vi "subBuildXYGraph.vi"(7 "Enable":bool=TRUE, 8 "error in (no error)":errorcluster, 9 "Reset":bool, 10 "Y Input":dynamicdata(waveform), 11 "X Input":dynamicdata(waveform)) -> (0 "error out":errorcluster, 2 "XY Graph":cluster{"X":dbl[], "Y":dbl[]}[](array[cluster]))   [LabVIEW 2020]
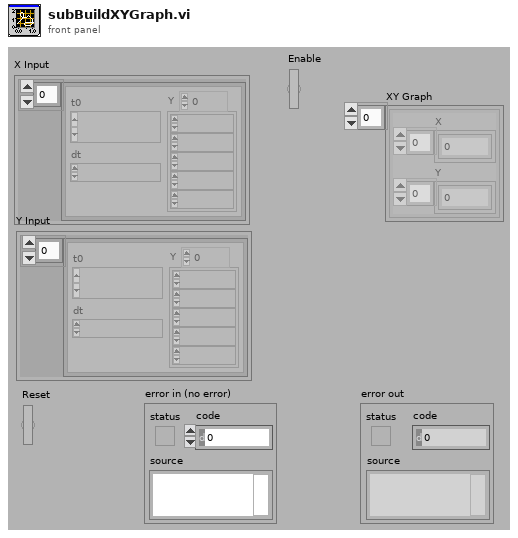
[diagram p1: front panel]
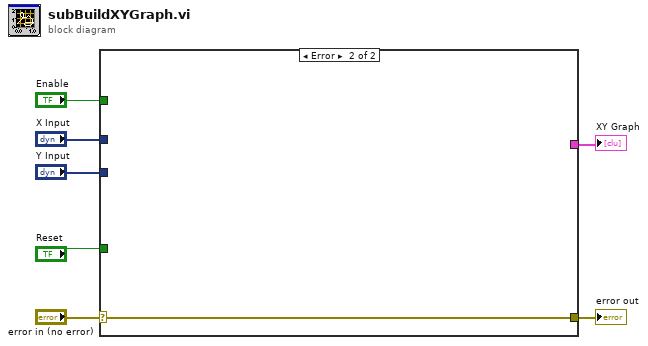
[diagram p0: block diagram]
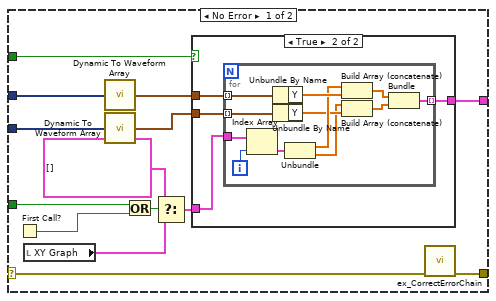
[diagram p2: hidden frame]
diagram:
  n1 = case shown="Error" "error in (no error)" {
    selector: "error in (no error)" -> [w9 w39]
    tunnel: [w21 _] -> w7
    tunnel: "Enable" -> [w18 _]
    tunnel: "Reset" -> [w16 _]
    tunnel: "Y Input" -> [w12 _]
    tunnel: "X Input" -> [w11 _]
    tunnel: [w10 w39] -> w1
    frame No Error {
      n2 = First Call?() -> (First Call?: T/F=w15:bool)
      n3 = local read "XY Graph"() -> (w8:cluster{"X":dbl[], "Y":dbl[]}[])
      n4 = call "Dynamic To Waveform Array.vi"("Input"=w11) -> ("Output"=w14:waveform(dbl)[])  [unwired: 4 out]
      n5 = call "Dynamic To Waveform Array.vi"("Input"=w12) -> ("Output"=w13:waveform(dbl)[])  [unwired: 4 out]
      n6 = Or(x=w16, y=w15) -> (x .or. y?=w17:bool)
      n7 = Select(t=cluster{"Y":dbl[], "Y":dbl[]}[] [] ("Output Array"), s=w17, f=w8) -> (s? t:f=w19:cluster{"X":dbl[], "Y":dbl[]}[])
      n8 = case shown="True" w18 {
        tunnel: [w22 w26] -> w21
        tunnel: w14 -> [_ w24]
        tunnel: w13 -> [_ w23]
        tunnel: w19 -> [w22 w25]
        frame False {
        }
        frame True {
          n9 = for {
            tunnel: [w38] -> w26 mode=indexing
            tunnel: w24 -> [w27] mode=indexing
            tunnel: w23 -> [w28] mode=indexing
            tunnel: w25 -> [w31]
            i -> [w29]
            n10 = Index Array(array=w31, index=w29) -> (element=w30:cluster{"X":dbl[], "Y":dbl[]})
            n11 = Unbundle By Name(w27) -> ("Y"=w37:dbl[])
            n12 = Unbundle By Name(w28) -> ("Y"=w34:dbl[])
            n13 = Unbundle(w30) -> ("X"=w35:dbl[], "Y"=w33:dbl[])
            n14 = Build Array (concatenate)(w35, w37) -> (w36:dbl[])
            n15 = Build Array (concatenate)(w33, w34) -> (w32:dbl[])
            n16 = Bundle(w36, w32) -> (w38:cluster{dbl[], dbl[]})  [unwired: 1 out]
          }
        }
      }
      n17 = call "ex_CorrectErrorChain.vi"("error in (no error)"=w9) -> ("error out"=w10:errorcluster)  [unwired: 1 in, 9 out]
    }
    frame Error {
    }
  }
  "XY Graph" <- w7
  "error out" <- w1
